vi "example1_17_09.vi"() -> ()   [LabVIEW 2025]
panel:
  in  "Numeric 2":dbl
  in  "Numeric1":dbl
  out "Soma ou Diferença":dbl
  in  "Boolean":bool
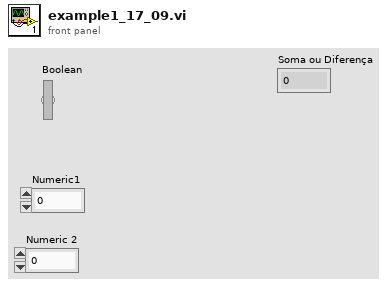
[diagram p1: front panel]
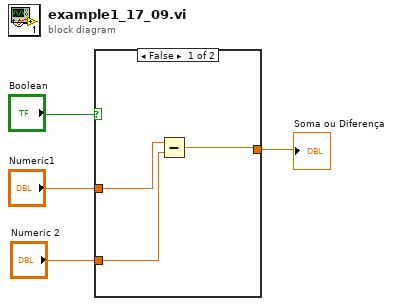
[diagram p0: block diagram]
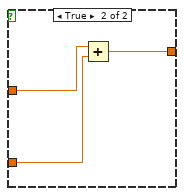
[diagram p2: hidden frame]
diagram:
  n1 = case shown="False" "Boolean" {
    tunnel: "Numeric1" -> [w7 w10]
    tunnel: "Numeric 2" -> [w6 w9]
    tunnel: [w5 w8] -> w1
    frame False {
      n2 = Subtract(x=w7, y=w6) -> (x-y=w5:dbl)
    }
    frame True {
      n3 = Add(x=w10, y=w9) -> (x+y=w8:dbl)
    }
  }
  "Soma ou Diferença" <- w1
